vi "Get ni_measurementlink_measurement_v1_GetMetadataResponse.vi"(8 "error in (no error)":errorcluster, 11 "gRPCid":T9) -> (0 "error out":errorcluster, 2 "package_templatemessage":T1, 3 "gRPCid out":T9)   [LabVIEW 2020, in "MeasurementTemplate_server.lvlib"]
uses:
  MeasurementTemplate_server.lvlib
  <vilib>/gRPC/LabVIEW gRPC Library/Shared/grpcId.ctl
  ni_measurementlink_measurement_v1_GetMetadataResponse.ctl
  ni_measurementlink_measurement_v1_MeasurementDetails.ctl
  ni_measurementlink_measurement_v1_MeasurementSignature.ctl
  ni_measurementlink_measurement_v1_ConfigurationParameter.ctl
  ni_measurementlink_measurement_v1_ConfigurationParameter_AnnotationsEntry.ctl
  google_protobuf_Any.ctl
  ni_measurementlink_measurement_v1_Output.ctl
  ni_measurementlink_measurement_v1_UserInterfaceDetails.ctl
  a51dd2a7-b5c1-4c09-9df4-8cd9d3bd0c19.vi
  <vilib>/gRPC/LabVIEW gRPC Library/Shared/TranslateGrpcError.vi
  <vilib>/AdvancedString/1D String Array to Delimited String.vi
  <vilib>/gRPC/LabVIEW gRPC Library/Server API/Server/Get Server DLL Path.vi
  <vilib>/gRPC/LabVIEW gRPC Library/grpc-lvsupport-release.lvlib
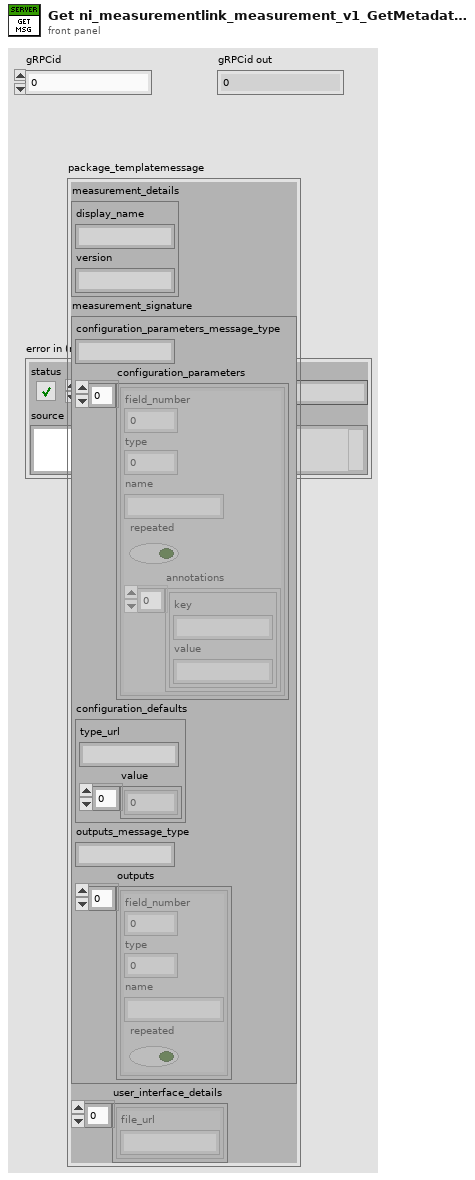
[diagram p1: front panel]
types:
  T1 = typedef "MeasurementTemplate_server.lvlib/ni_measurementlink_measurement_v1_GetMetadataResponse.ctl" = cluster{"measurement_details":T2, "measurement_signature":T3, "user_interface_details":T8[]}
  T2 = typedef "MeasurementTemplate_server.lvlib/ni_measurementlink_measurement_v1_MeasurementDetails.ctl" = cluster{"display_name":string, "version":string}
  T3 = typedef "MeasurementTemplate_server.lvlib/ni_measurementlink_measurement_v1_MeasurementSignature.ctl" = cluster{"configuration_parameters_message_type":string, "configuration_parameters":T4[], "configuration_defaults":T6, "outputs_message_type":string, "outputs":T7[]}
  T4 = typedef "MeasurementTemplate_server.lvlib/ni_measurementlink_measurement_v1_ConfigurationParameter.ctl" = cluster{"field_number":i32, "type":i32, "name":string, "repeated":bool, "annotations":T5[]}
  T5 = typedef "MeasurementTemplate_server.lvlib/ni_measurementlink_measurement_v1_ConfigurationParameter_AnnotationsEntry.ctl" = cluster{"key":string, "value":string}
  T6 = typedef "MeasurementTemplate_server.lvlib/google_protobuf_Any.ctl" = cluster{"type_url":string, "value":u8[]}
  T7 = typedef "MeasurementTemplate_server.lvlib/ni_measurementlink_measurement_v1_Output.ctl" = cluster{"field_number":i32, "type":i32, "name":string, "repeated":bool}
  T8 = typedef "MeasurementTemplate_server.lvlib/ni_measurementlink_measurement_v1_UserInterfaceDetails.ctl" = cluster{"file_url":string}
  T9 = typedef "grpc-lvsupport-release.lvlib/grpcId.ctl" = u64
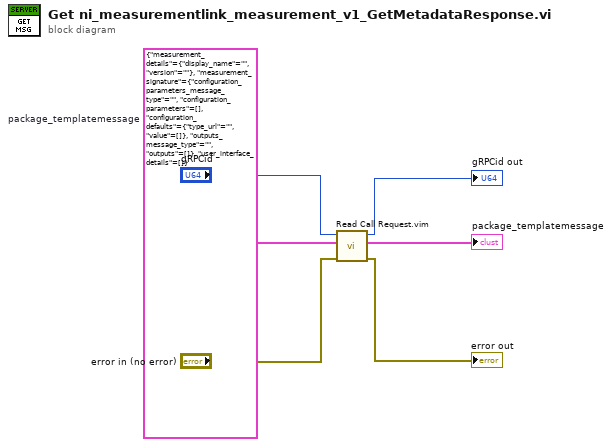
[diagram p0: block diagram]
diagram:
  w2 = T1 {"measurement_details"={"display_name"="", "version"=""}, "measurement_signature"={"configuration_parameters_message_type"="", "configuration_parameters"=[], "configuration_defaults"={"type_url"="", "value"=[]}, "outputs_message_type"="", "outputs"=[]}, "user_interface_details"=[]}  # package_templatemessage
  n1 = call "Read Call Request.vim"("error in"="error in (no error)", "Request Type"=w2, "gRPCid in"="gRPCid") -> ("error out"=→"error out":errorcluster, "Request Data"=→"package_templatemessage":T1, "gRPCid out"=→"gRPCid out":T9)  [unwired: 6 in]
